vi "ziError.vi"(0 "Conn":u64 format="0x%08x", 1 "ziErrorCode":u32, 3 "Error In":errorcluster, 4 "Annotation":string) -> (6 "Error Out":errorcluster)   [LabVIEW 2016, in "Zurich Instruments LabOne.lvlib"]
uses:
  Zurich Instruments LabOne.lvlib
  <vilib>/Utility/error.llb/DialogType.ctl
  Zurich Instruments/LabOne/API/LabVIEW/Zurich Instruments LabOne/Private/ziLV64.framework
panel:
  in  "Caller 2":string
  out "Severity":enum16{"Info", "Warning", "Error"}(ring)
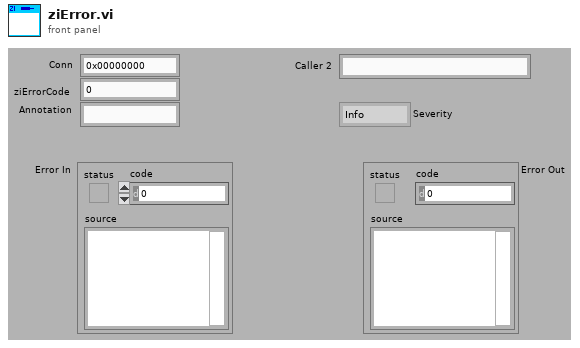
[diagram p1: front panel]
types:
  T1 = typedef "DialogType.ctl" = u16
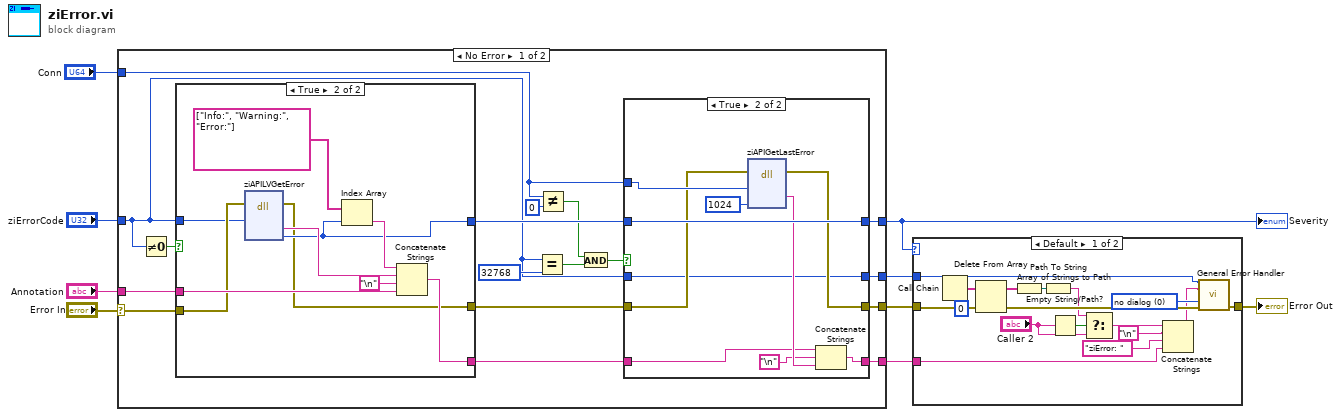
[diagram p0: block diagram]
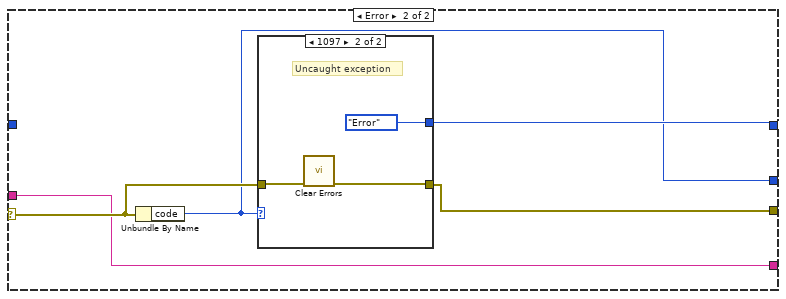
[diagram p5: hidden frame]
diagram:
  n1 = case shown="No Error" "Error In" {
    selector: "Error In" -> [w24 w56]
    tunnel: [w22 w55] -> w5
    tunnel: "ziErrorCode" -> [w14 _]
    tunnel: "Annotation" -> [w25 w53]
    tunnel: [w19 w54] -> w6
    tunnel: [w21 w53] -> w4
    tunnel: [w18 w52] -> w3
    tunnel: "Conn" -> [w10 _]
    frame No Error {
      n2 = Not Equal To 0?(x=w14) -> (x != 0?=w26:bool)
      n3 = case shown="True" w26 {
        tunnel: [w41 w42] -> w23
        tunnel: w24 -> [w41 w47]
        tunnel: w14 -> [_ w43]
        tunnel: w25 -> [_ w48]
        tunnel: [_ w45] -> w17
        tunnel: [_ w44] -> w20
        frame False {
        }
        frame True {
          n4 = dll-call lib="Users/arkady/Desktop/ado/github/resonant_ultrasound_arxiv/maglab ultrasound -- arkady --arxiv/Zurich Instruments/LabOne/API/LabVIEW/Zurich Instruments LabOne/Private/ziLV*.*" fn="ziAPILVGetError" label="ErrorMsg"(error in=w47, "Status"=w43) -> (error out=w42:errorcluster, "ErrorMessage"=w49:string, "Severity"=w45:u32)  [unwired: 3 in, 4 out]
          n5 = Index Array(array=string[] ["Info:", "Warning:", "Error:"], index=w45) -> (element=w51:string)
          n6 = Concatenate Strings(w51, w49, "\n", w48) -> (w44:string)
        }
      }
      n7 = Equal?(x=w14, y=u32 32768) -> (x = y?=w16:bool)
      n8 = Not Equal?(x=w10, y=u64 0 ("Conn 2")) -> (x != y?=w12:bool)
      n9 = And(x=w12, y=w16) -> (x .and. y?=w13:bool)
      n10 = case shown="True" w13 {
        tunnel: w17 -> [w30 w40]
        tunnel: [w30 w40] -> w19
        tunnel: w23 -> [w29 w37]
        tunnel: [w29 w36] -> w22
        tunnel: [w28 w34] -> w21
        tunnel: w20 -> [w28 w33]
        tunnel: [w27 w31] -> w18
        tunnel: w10 -> [_ w38]
        tunnel: w14 -> [w27 w31]
        frame False {
        }
        frame True {
          n11 = dll-call lib="Users/arkady/Desktop/ado/github/resonant_ultrasound_arxiv/maglab ultrasound -- arkady --arxiv/Zurich Instruments/LabOne/API/LabVIEW/Zurich Instruments LabOne/Private/ziLV*.*" fn="ziAPIGetLastError"(error in=w37, "conn"=w38, "buffer"=u32 1024) -> (error out=w36:errorcluster, "ErrorMessage"=w35:string)  [unwired: 3 in, 4 out]
          n12 = Concatenate Strings(w33, "\n", w35) -> (w34:string)
        }
      }
    }
    frame Error {
      n13 = Unbundle By Name(w56) -> ("code"=w52:i32)
      n14 = case shown="1097" w52 {
        tunnel: w56 -> [w57 w59]
        tunnel: [w57 w58] -> w55
        tunnel: [_ enum16{"Info", "Warning", "Error"}."Error" ("Severity")] -> w54
        frame 0, Default {
        }
        frame 1097 {
          # "Uncaught exception"
          n15 = call <vilib>:"Clear Errors.vi"("error in (no error)"=w59) -> ("error out"=w58:errorcluster)  [unwired: 5 in, 1 out]
        }
      }
    }
  }
  "Severity" <- w6
  n16 = case shown="Default" w6 {
    tunnel: w5 -> [w75 w77]
    tunnel: [w74 w77] -> w2
    tunnel: w3 -> [w73 _]
    tunnel: w4 -> [w69 _]
    frame Default {
      w76 = T1 0 items=["no dialog", "OK message", "continue or stop message", "OK message + warnings", "continue/stop + warnings"] ("type of dialog (OK msg:1)")
      n17 = Call Chain() -> (call chain=w63:string[])
      n18 = Delete From Array(array=w63, index=0) -> (array with subset deleted=w62:string[])  [unwired: 1 in, 1 out]
      n19 = Array of Strings to Path(0:w62) -> (2:w66:path)  [unwired: 1 out]
      n20 = Path To String(path=w66) -> (string=w65:string)
      n21 = Empty String/Path?(string/path="Caller 2") -> (empty?=w68:bool)
      n22 = Select(t=w65, s=w68, f="Caller 2") -> (s? t:f=w64:string)
      n23 = Concatenate Strings(w64, "\n", "ziError: " ("string"), w69) -> (w70:string)
      n24 = call <vilib>:"General Error Handler.vi"("[error code] (0)"=w73, "[error source] (\" \")"=w70, "type of dialog (OK msg:1)"=w76, "error in (no error)"=w75) -> ("error out"=w74:errorcluster)  [unwired: 3 in, 8 out]
    }
    frame 0 {
    }
  }
  "Error Out" <- w2
